vi "Get First.vi"(8 "error in (no error)":errorcluster caption="错误输入（无错误）", 11 "Iterator(Abstract) 输入":refnum<class "具体迭代器.lvclass"> caption="DNL_LabVIEW Object in") -> (0 "error out":errorcluster caption="错误输出", 2 "LabVIEW对象":refnum<class>, 3 "Iterator(Abstract) 输出":refnum<class "具体迭代器.lvclass"> caption="DNL_LabVIEW Object out")   [LabVIEW 2011, in "迭代器.lvlib" / "具体迭代器.lvclass"]
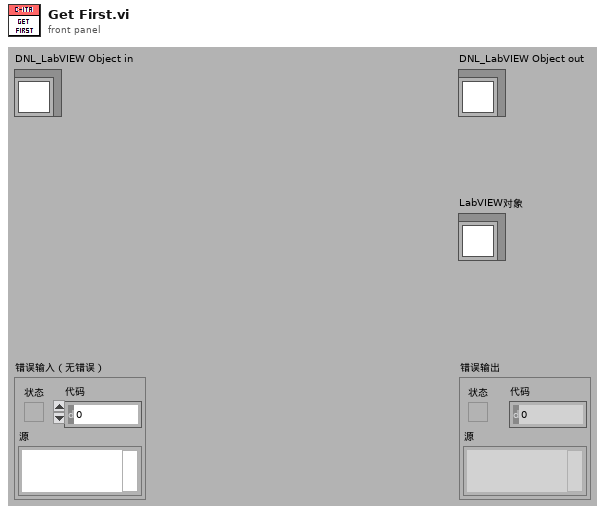
[diagram p1: front panel]
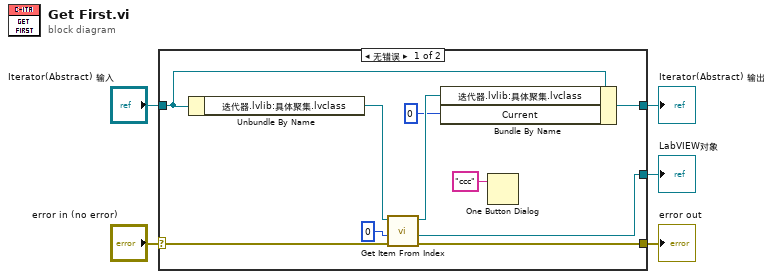
[diagram p0: block diagram]
diagram:
  n1 = case shown="无错误" "error in (no error)" {
    selector: "error in (no error)" -> [w10 w17]
    tunnel: [w9 w17] -> w4
    tunnel: "Iterator(Abstract) 输入" -> [w14 w16]
    tunnel: [w12 w16] -> w2
    tunnel: [w11 _] -> w1
    frame No Error {
      n2 = Unbundle By Name(w14) -> ("迭代器.lvlib:具体聚集.lvclass"=w15:refnum<class "具体聚集.lvclass">)
      n3 = call "Get Item From Index.vi"("error in (no error)"=w10, "Index"=0, "具体聚集 输入"=w15) -> ("error out"=w9:errorcluster, "迭代器.lvlib:雇员.lvclass"=w11:refnum<class "雇员.lvclass">, "具体聚集 输出"=w13:refnum<class "具体聚集.lvclass">)  [unwired: 6 in]
      n4 = Bundle By Name(cluster=w14, "迭代器.lvlib:具体聚集.lvclass"=w13, "Current"=0) -> (w12:refnum<class "具体迭代器.lvclass">)
      n5 = One Button Dialog(message="ccc" ("消息")) -> ()  [unwired: 1 in, 1 out]
    }
    frame Error {
    }
  }
  "error out" <- w4
  "Iterator(Abstract) 输出" <- w2
  "LabVIEW对象" <- w1
